vi "token.valid.vi"(8 "error in":errorcluster, 11 "token":path) -> (0 "error out":errorcluster, 3 "valid":bool)   [LabVIEW 2024, in "nominal labview client.lvlib"]
uses:
  nominal labview client.lvlib
  <vilib>/Nominal/Nominal IO Client/Nominal Client/Nominal Client.lvclass/Nominal Client.ctl
  33f66643-65c2-4a5e-bbae-ec423fb1ee78.vi
  <vilib>/Nominal/Nominal IO Client/Nominal Client/private_data.set.vi
  <vilib>/Utility/error.llb/Error Cluster From Error Code.vi
  <vilib>/addons/_JKI.lib/REST Client/classes/REST Client/Create REST Client.vi
  <vilib>/Nominal/Nominal IO Client/Nominal Client/Nominal Client.lvclass
  <vilib>/addons/_JKI.lib/REST Client/classes/REST Client/REST Client.lvclass
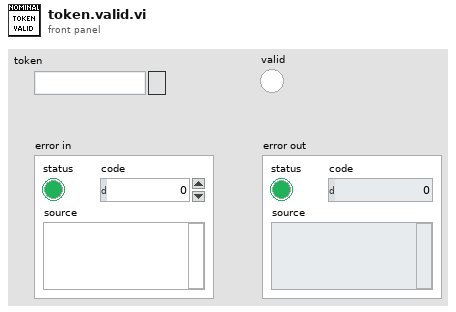
[diagram p1: front panel]
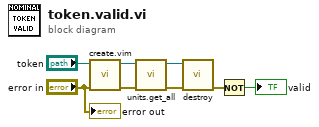
[diagram p0: block diagram]
diagram:
  n1 = call "create.vim"("error in"="error in", "API Token (string or path)"="token") -> ("error out"=w2:errorcluster, "Nominal Client"=w5:refnum<class "Nominal Client.lvclass">)  [unwired: 8 in]
  n2 = call <vilib>:"units.get_all.vi"("error in"=w2, "Nominal Client in"=w5) -> ("error out"=w3:errorcluster, "Nominal Client out"=w4:refnum<class "Nominal Client.lvclass">)  [unwired: 7 in, 1 out]
  n3 = call <vilib>:"destroy.vi"("error in"=w3, "Nominal Client"=w4) -> ("error out"=w1:errorcluster)  [unwired: 9 in]
  n4 = Not(x=w1) -> (.not. x?=→"valid":bool)
  "error out" <- "error in"
